vi "changeSummaryState.vi"(8 "error in (no error)":errorcluster, 10 "newSummaryState":T1, 11 "Model in":refnum<class "Model.lvclass">) -> (0 "error out":errorcluster, 3 "Model out":refnum<class "Model.lvclass">)   [LabVIEW 2012, in "Model.lvclass"]
doc: "Changes the summary state to the value of newSummaryState and publishes the new state."
uses:
  Model.lvclass
  C/Program Files (x86)/National Instruments/LabVIEW 2012/user.lib/Common/ComponentModel/ComponentModel/Typedefs/ComponentStateValues.ctl
  Typedefs/PubDataSV.ctl
  Model.lvclass/Model.ctl
  Typedefs/EXATypedefs.lvlib
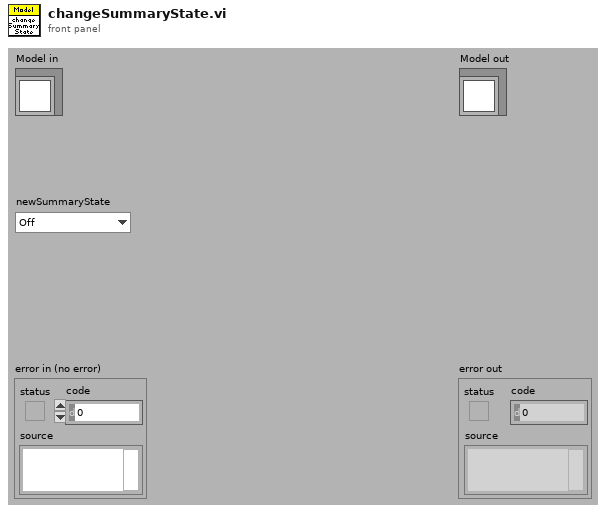
[diagram p1: front panel]
types:
  T1 = typedef "componentStateValues.ctl" = enum16{"Off", "Standby", "Enabled", "Disabled", "Fault"}
  T2 = typedef "EXATypedefs.lvlib/PubDataSV.ctl" = enum16{"DetailedState", "ErrorCode", "Heartbeat", "LoopTime_ms", "LoopTimeOutOfRange", "SummaryState", "Timestamp"}
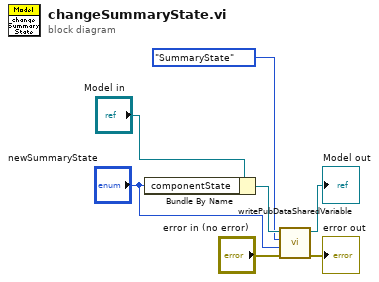
[diagram p0: block diagram]
diagram:
  n1 = Bundle By Name(cluster="Model in", "componentState"="newSummaryState") -> (w6:refnum<class "Model.lvclass">)
  n2 = call "writePubDataSharedVariable.vi"("error in (no error)"="error in (no error)", "value"="newSummaryState", "pubDataSV"=PubDataSV."SummaryState" ("PubDataSV"), "Model in"=w6) -> ("error out"=→"error out":errorcluster, "Model out"=→"Model out":refnum<class "Model.lvclass">)  [unwired: 6 in]
